vi "Read FitCoeff.vi"(8 "error in (no error)":errorcluster, 11 "CRDS Cell Data in":refnum<class "CRDS Cell Data.lvclass">) -> (0 "error out":errorcluster, 2 "FitCoeff":dbl[](array[numeric]), 3 "CRDS Cell Data out":refnum<class "CRDS Cell Data.lvclass">)   [LabVIEW 2019, in "CRDS Cell Data.lvclass"]
uses:
  CRDS Cell Data.lvclass
  CRDS Cell Data.lvclass/CRDS Cell Data.ctl
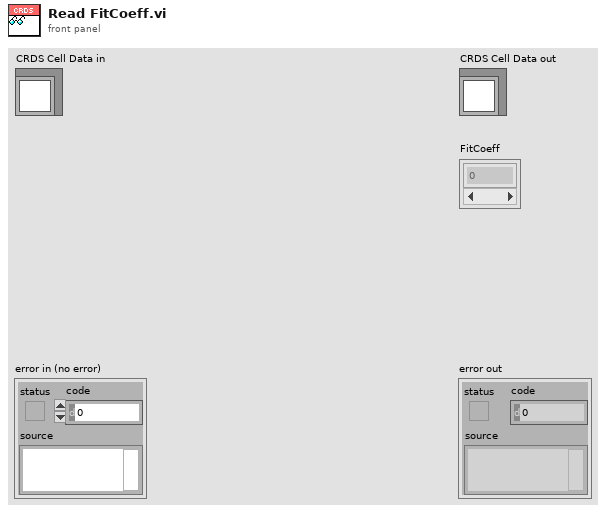
[diagram p1: front panel]
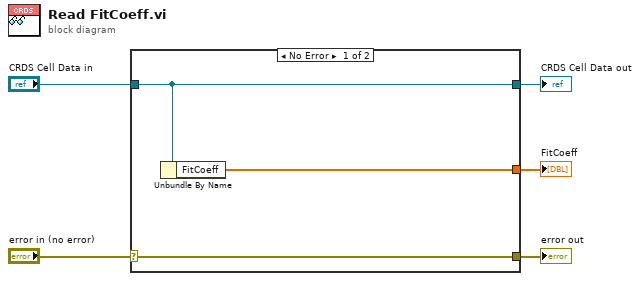
[diagram p0: block diagram]
diagram:
  n1 = case shown="No Error" "error in (no error)" {
    selector: "error in (no error)" -> [w8 w9]
    tunnel: [w8 w9] -> w4
    tunnel: [w7 w10] -> w2
    tunnel: "CRDS Cell Data in" -> [w7 w10]
    tunnel: [w6 _] -> w1
    frame No Error {
      n2 = Unbundle By Name(w7) -> ("FitCoeff"=w6:dbl[])
    }
    frame Error {
    }
  }
  "error out" <- w4
  "CRDS Cell Data out" <- w2
  "FitCoeff" <- w1
